vi "Pic Overlay i Box.vi"(8 "error in (no error)":errorcluster, 10 "Picture in":picture, 11 "LF2R IDE in":refnum<class "Main Panel.lvclass">) -> (0 "error out":errorcluster, 2 "Picture out":picture, 3 "LF2R IDE out":refnum<class "Main Panel.lvclass">)   [LabVIEW 2018, in "Main Panel.lvlib" / "Main Panel.lvclass"]
uses:
  Main Panel.lvclass
  Main Panel.lvclass/Main Panel.ctl
  Picture Process/Picture Process.lvclass
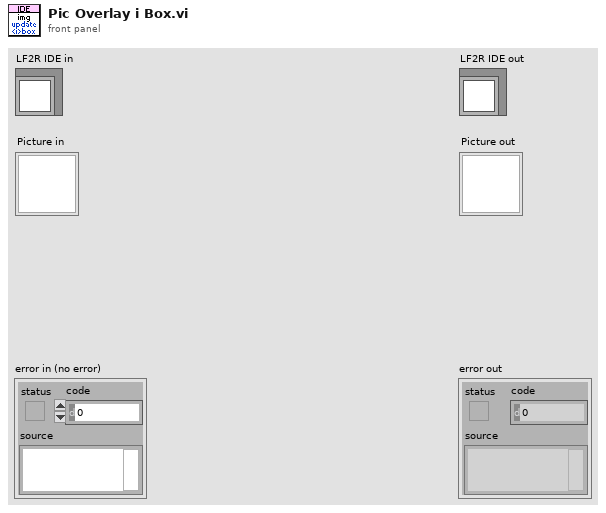
[diagram p1: front panel]
types:
  T1 = typedef "Data Parser.lvclass/frame i data.ctl" = cluster{"kind":string, "x":string, "y":string, "w":string, "h":string, "dvx":string, "dvy":string, "dvz":string, "fall":string, "arest":string, "vrest":string, "bdefend":string, "injury":string, "zwidth":string, "effect":string, "catchingact":string, "caughtact":string}
  T2 = cluster{"Fill Color":u32, "Border Color":u32, "Show?":bool}
  T3 = cluster{"x":string, "y":string, "w":string, "h":string}
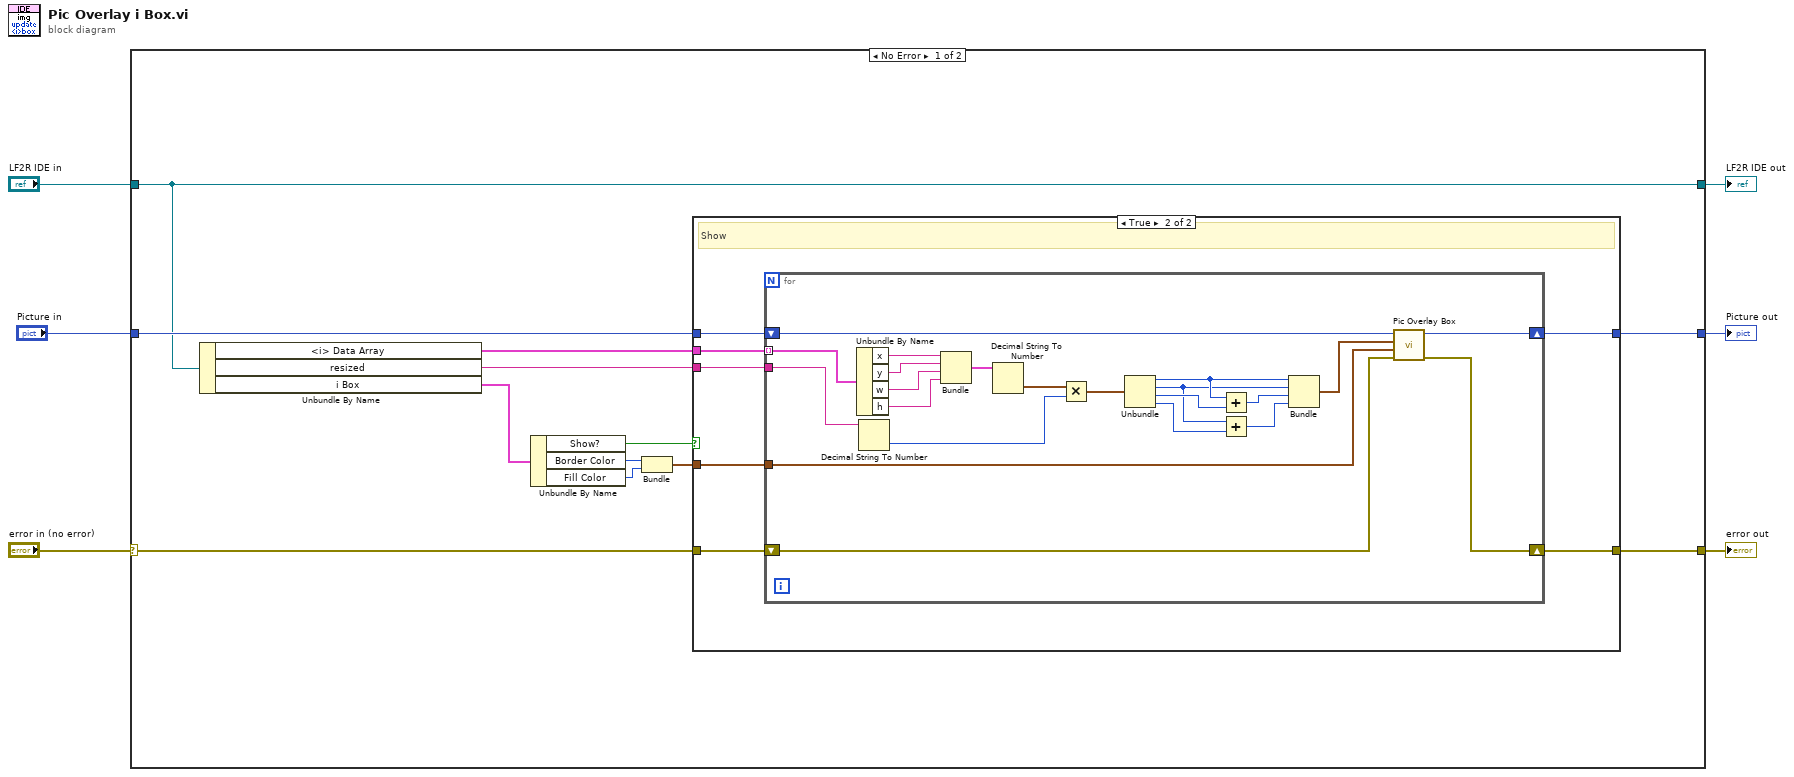
[diagram p0: block diagram]
diagram:
  n1 = case shown="No Error" "error in (no error)" {
    selector: "error in (no error)" -> [w17 w52]
    tunnel: [w16 w52] -> w5
    tunnel: [w7 w51] -> w3
    tunnel: "LF2R IDE in" -> [w7 w51]
    tunnel: "Picture in" -> [w9 w50]
    tunnel: [w8 w50] -> w1
    frame No Error {
      n2 = Unbundle By Name(w7) -> ("<i> Data Array"=w18:T1[], "resized"=w15:string, "i Box"=w14:T2)
      n3 = Unbundle By Name(w14) -> ("Show?"=w13:bool, "Border Color"=w12:u32, "Fill Color"=w11:u32)
      n4 = Bundle("Border Color"=w12, "Fill Color"=w11) -> (w10:cluster{"Border Color":u32, "Fill Color":u32})  [unwired: 1 in]
      n5 = case shown="True" w13 {
        tunnel: w18 -> [_ w27]
        tunnel: w17 -> [w20 w26]
        tunnel: [w20 w21] -> w16
        tunnel: w15 -> [_ w25]
        tunnel: w10 -> [_ w24]
        tunnel: w9 -> [w19 w23]
        tunnel: [w19 w22] -> w8
        frame False {
          # "Skip"
        }
        frame True {
          # "Show"
          n6 = for {
            tunnel: w27 -> [w49] mode=indexing
            shift-right: [w28] -> w21
            shift-left: w26 -> [w29]
            shift-right: [w32] -> w22
            shift-left: w23 -> [w33]
            tunnel: w25 -> [w35]
            tunnel: w24 -> [w30]
            n7 = Unbundle By Name(w49) -> ("x"=w46:string, "y"=w45:string, "w"=w44:string, "h"=w43:string)
            n8 = Decimal String To Number(string=w35) -> (number=w34:i32)  [unwired: 2 in, 1 out]
            n9 = Bundle("x"=w46, "y"=w45, "w"=w44, "h"=w43) -> (w42:T3)  [unwired: 1 in]
            n10 = Decimal String To Number(string=w42) -> (number=w37:cluster{"x":i32, "y":i32, "w":i32, "h":i32})  [unwired: 2 in, 1 out]
            n11 = Multiply(x=w37, y=w34) -> (x*y=w36:cluster{"x":i32, "y":i32, "w":i32, "h":i32})
            n12 = Unbundle(w36) -> ("x"=w41:i32, "y"=w39:i32, "w"=w40:i32, "h"=w38:i32)
            n13 = Add(x=w41, y=w40) -> (x+y=w48:i32)
            n14 = Add(x=w39, y=w38) -> (x+y=w47:i32)
            n15 = Bundle("x"=w41, "y"=w39, w48, w47) -> (w31:cluster{"x":i32, "y":i32, i32, i32})  [unwired: 1 in]
            n16 = call "Pic Overlay Box.vi"("error in (no error)"=w29, "Color"=w30, "Rectangle"=w31, "Picture in"=w33) -> ("error out"=w28:errorcluster, "Picture out"=w32:picture)  [unwired: 6 in]
          }
        }
      }
    }
    frame Error {
    }
  }
  "error out" <- w5
  "LF2R IDE out" <- w3
  "Picture out" <- w1
